vi "browseVariant.vi"(4 "Variant":variant caption="Value", 5 "Name":string, 6 "error in (no error)":errorcluster, 7 "ParentTag":string, 9 "VariantProbe.lvclass in":refnum<class "VariantTree__VP.lvclass">) -> (0 "error out":errorcluster, 3 "VariantProbe.lvclass out":refnum<class "VariantTree__VP.lvclass">)   [LabVIEW 2011, in "VariantTree__VP.lvclass"]
uses:
  VariantTree__VP.lvclass
  VariantTree__VP.lvclass/VariantTree__VP.ctl
  <vilib>/Utility/VariantDataType/VariantType.lvlib
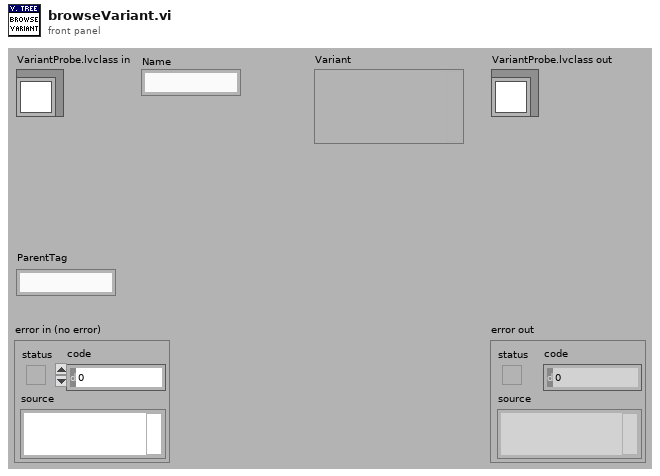
[diagram p1: front panel]
types:
  T1 = typedef "Type Descriptor Enumeration__ogtk.ctl" = enum8{"<Null>", "I8", "I16", "I32", "I64", "U8", "U16", "U32", "U64", "SGL", "DBL", "EXT", "CSG", "CDB", "CXT", "0x0F", "0x10", "0x11", "0x12", "0x13", "0x14", "Enum U8", "Enum U16", "Enum U32", "Enum U64", "SGL PQ", "DBL PQ", "EXT PQ", "CSG PQ", "CDB PQ", "CXT PQ", "0x1F", "0x20", "Boolean", "0x22", "0x23", "0x24", "0x25", "0x26", "0x27", "0x28", "0x29", "0x2A", "0x2B", "0x2C", "0x2D", "0x2E", "0x2F", "String", "0x31", "Path", "Pict", "0x34", "0x35", "0x36", "DAQ", "0x38", "0x39", "0x3A", "0x3B", "0x3C", "0x3D", "0x3E", "0x3F", "Array", "0x41", "0x42", "0x43", "0x44", "0x45", "0x46", "0x47", "0x48", "0x49", "0x4A", "0x4B", "0x4C", "0x4D", "0x4E", "0x4F", "Cluster", "0x51", "0x52", "Variant", "Waveform", "0x55", "0x56", "0x57", "0x58", "0x59", "0x5A", "0x5B", "0x5C", "0x5D", "0x5E", "0x5F", "0x60", "0x61", "0x62", "0x63", "0x64", "0x65", "0x66", "0x67", "0x68", "0x69", "0x6A", "0x6B", "0x6C", "0x6D", "0x6E", "0x6F", "Refnum"}
  T2 = typedef "Type Descriptor Header__ogtk.ctl" = cluster{"length":u16, "private":u8, "type":T1, "# elements":u16}
  T3 = typedef "Physical Units__ogtk.ctl" = cluster{"Base Units":enum16{"radian", "steradian", "second", "meter", "kilogram", "ampere", "kelvin", "mole", "candela"}, "Exponent":i16}
  T4 = enum16{"radian", "steradian", "second", "meter", "kilogram", "ampere", "kelvin", "mole", "candela"}
  T5 = typedef "VariantType.lvlib/RefnumType.ctl" = enum16{"NotARefnum", "UnknownRefnum", "Generic", "Datalog", "ByteStream", "Device", "Occurence", "TCPNetConnection", "Auto", "Menu", "Imaq", "Hardware", "DataSocket", "Visa", "IVI", "UDPNetConnection", "Notifier", "Queue", "Irda", "EventReg", "DotNet", "UserEvent", "Callback", "UNUSED_EMPTY_POSITION", "BlueToothNetConnection", "LVObjApp", "LVObjVI", "LVObjUnknown", "GenericClass", "UserDefinedRefnumTag", "DataValue"}
  T6 = enum32{"invalid VI type", "Standard VI", "Control VI", "Global VI", "Polymorphic VI", "Configuration VI", "SubSystem", "Facade VI", "Method VI", "Statechart Diagram VI"}
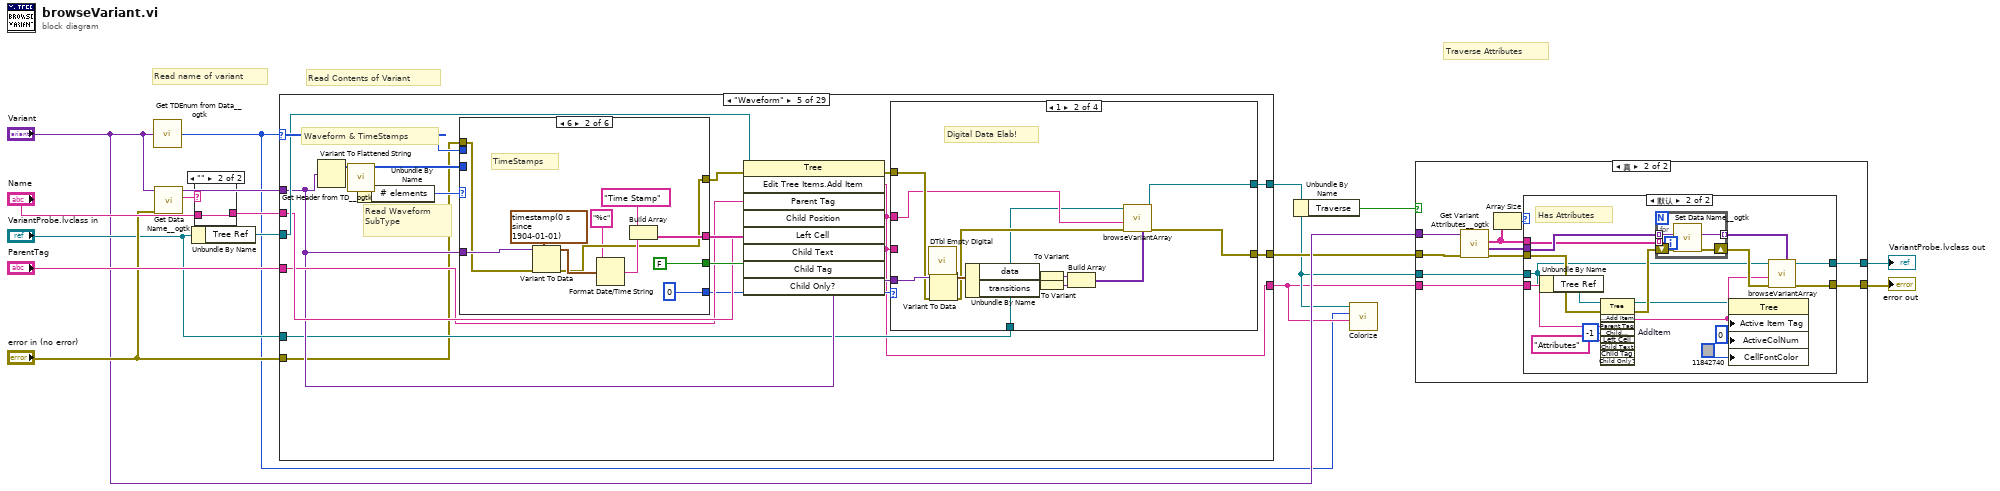
[diagram p0: block diagram]
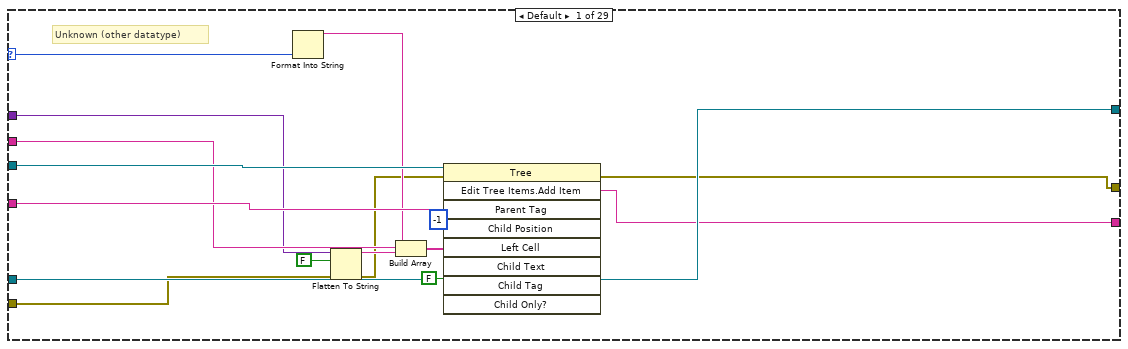
[diagram p5: hidden frame]
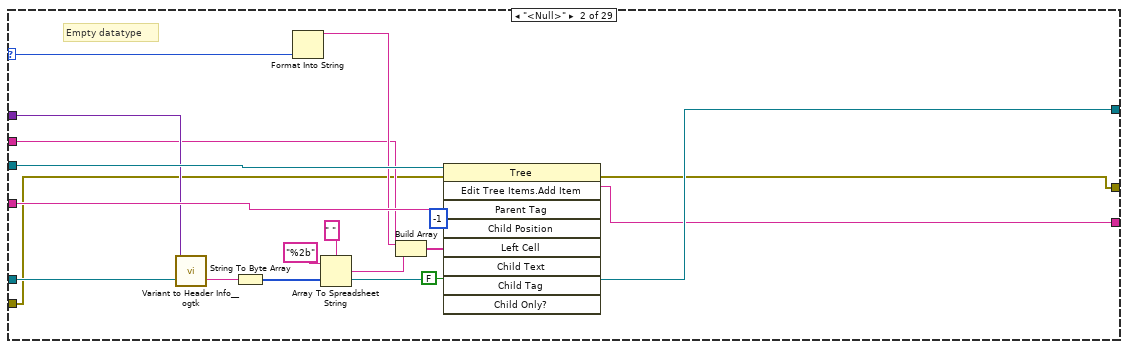
[diagram p6: hidden frame]
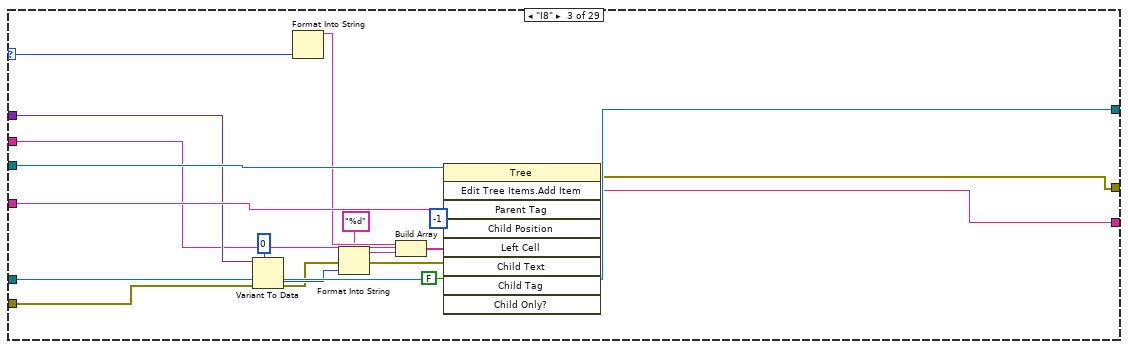
[diagram p7: hidden frame]
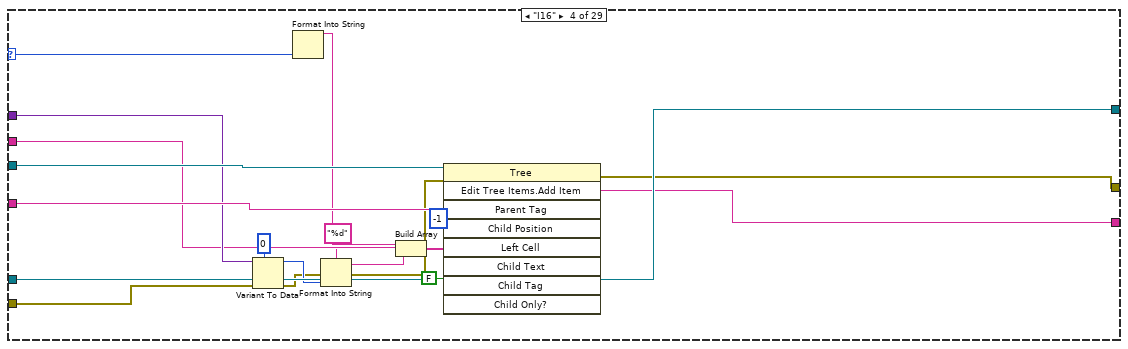
[diagram p8: hidden frame]
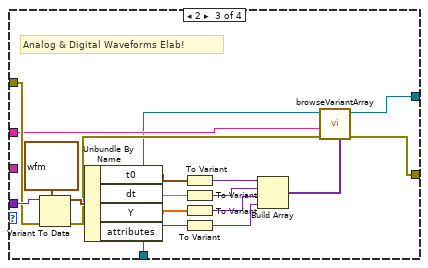
[diagram p10: hidden frame]
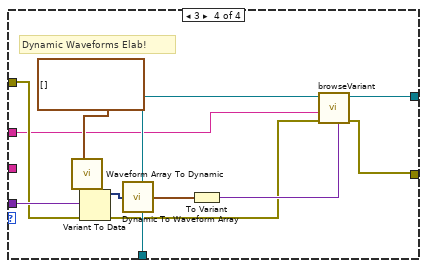
[diagram p11: hidden frame]
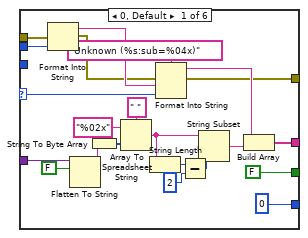
[diagram p12: hidden frame]
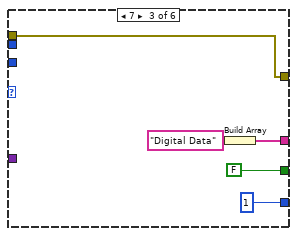
[diagram p13: hidden frame]
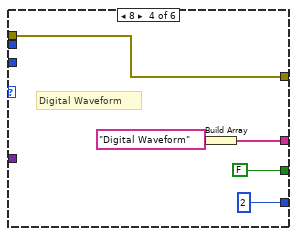
[diagram p14: hidden frame]
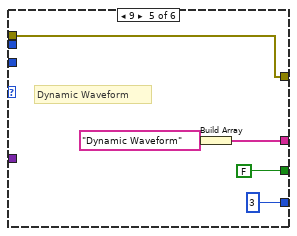
[diagram p15: hidden frame]
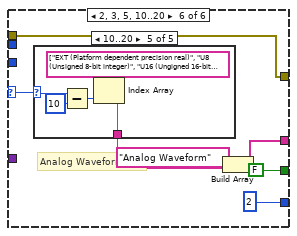
[diagram p16: hidden frame]
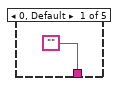
[diagram p17: hidden frame]
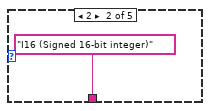
[diagram p18: hidden frame]
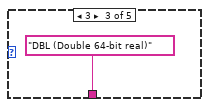
[diagram p19: hidden frame]
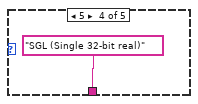
[diagram p20: hidden frame]
diagram:
  # "Traverse Attributes"
  # "Read Contents of Variant"
  # "Read name of variant"
  n1 = call <userlib>:"Get TDEnum from Data__ogtk.vi"("Data"="Variant") -> ("Type Descriptor Enumeration"=w1:T1)  [unwired: 4 in]
  n2 = call <userlib>:"Get Data Name__ogtk.vi"("error in (no error)"="error in (no error)", "Data"="Variant") -> ("Data Name"=w16:string, "Data dup"=w14:variant)  [unwired: 7 in, 1 out]
  n3 = Unbundle By Name("VariantProbe.lvclass in") -> ("Tree Ref"=w4:refnum<vi>)
  n4 = case shown="\"\"" w16 {
    selector: w16 -> [w17 _]
    tunnel: [w17 w18] -> w13
    tunnel: "Name" -> [_ w18]
    frame Default {
    }
    frame "" {
    }
  }
  n5 = case shown="\"Waveform\"" w1 {
    selector: w1 -> [w34 w52 w71 w90 w105 w237 w256 w275 w294 w313 w332 w350 w368 w386 w404 w422 w440 w463 w497 w531 w565 w591 w607 w624 w640 _ _ _ w711]
    tunnel: w14 -> [w25 w41 w64 w83 w97 w230 w249 w268 w287 w306 w325 w339 w358 w376 w394 w412 w430 w468 w485 w519 w553 w580 w598 w615 w631 w652 w666 w696 w702]
    tunnel: w4 -> [w31 w49 w68 w87 w104 w234 w253 w272 w291 w310 w329 w347 w365 w383 w401 w419 w437 w467 w494 w528 w562 w588 w604 w621 w637 w662 w677 w701 w709]
    tunnel: "ParentTag" -> [w33 w51 w70 w89 w99 w236 w255 w274 w293 w312 w331 w349 w367 w385 w403 w421 w439 w466 w496 w530 w564 w590 w606 w623 w639 w661 w676 w700 w710]
    tunnel: w13 -> [w26 w40 w63 w82 w100 w229 w248 w267 w286 w305 w324 w340 w357 w375 w393 w411 w429 w449 w488 w522 w556 w579 w599 w614 w632 w653 w673 w695 w707]
    tunnel: "VariantProbe.lvclass in" -> [w23 w38 w61 w80 w96 w227 w246 w265 w284 w303 w322 w337 w355 w373 w391 w409 w427 w445 w478 w512 w546 w577 w596 w612 w629 w643 w671 w690 w706]
    tunnel: [w23 w38 w61 w80 w95 w227 w246 w265 w284 w303 w322 w337 w355 w373 w391 w409 w427 w445 w478 w512 w546 w577 w596 w612 w629 w642 w670 w688 w706] -> w3
    tunnel: "error in (no error)" -> [w22 w37 w59 w78 w94 w226 w244 w264 w283 w301 w321 w335 w354 w372 w390 w408 w425 w444 w477 w511 w545 w575 w594 w609 w628 w649 w668 w693 _]
    tunnel: [w20 w36 w60 w79 w92 w225 w245 w263 w282 w302 w314 w334 w352 w370 w388 w406 w424 w442 w472 w506 w540 w574 w593 w611 w626 w646 w669 w692 w705] -> w8
    tunnel: [w19 w35 w53 w72 w91 w219 w238 w257 w276 w295 w315 w333 w351 w369 w387 w405 w423 w441 w471 w505 w539 w573 w592 w608 w625 w641 w667 w687 w704] -> w2
    frame Default {
      # "Unknown (other datatype)"
      n6 = Format Into String(w34) -> (resulting string=w30:string)  [unwired: 3 in, 1 out]
      n7 = Flatten To String(anything=w25, prepend array or string size? (T)=FALSE, error in (no error)=w22) -> (data string=w28:string, error out=w21:errorcluster)  [unwired: 1 in, 1 out]
      n8 = Build Array(w30, w28) -> (w29:string[])
      n9 = invoke class="Tree" method="Edit Tree Items.Add Item"(reference=w31, error in=w21, "Parent Tag"=w33, "Child Position"=-1, "Left Cell"=w26, "Child Text"=w29, "Child Only?"=FALSE) -> (error out=w20:errorcluster, "Edit Tree Items:Add Item"=w19:string)  [unwired: 2 in, 7 out]
    }
    frame "<Null>" {
      # "Empty datatype"
      n10 = call <userlib>:"Variant to Header Info__ogtk.vi"("Variant"=w41) -> ("data string"=w43:string)  [unwired: 3 in, 2 out]
      n11 = String To Byte Array(string=w43) -> (unsigned byte array=w42:u8[])
      n12 = Format Into String(w52) -> (resulting string=w48:string)  [unwired: 3 in, 1 out]
      n13 = Array To Spreadsheet String(delimiter (Tab)=" ", array=w42, 3:"%2b" ("format string")) -> (spreadsheet string=w44:string)
      n14 = Build Array(w48, w44) -> (w47:string[])
      n15 = invoke class="Tree" method="Edit Tree Items.Add Item"(reference=w49, error in=w37, "Parent Tag"=w51, "Child Position"=-1, "Left Cell"=w40, "Child Text"=w47, "Child Only?"=FALSE) -> (error out=w36:errorcluster, "Edit Tree Items:Add Item"=w35:string)  [unwired: 2 in, 7 out]
    }
    frame "I8" {
      n16 = Variant To Data(error in=w59, type=i8 0, Variant=w64) -> (data=w58:i8, error out=w55:errorcluster)
      n17 = Format Into String(w71) -> (resulting string=w67:string)  [unwired: 3 in, 1 out]
      n18 = Format Into String(format string="%d", error in=w55, w58) -> (resulting string=w57:string, error out=w54:errorcluster)  [unwired: 1 in]
      n19 = Build Array(w67, w57) -> (w66:string[])
      n20 = invoke class="Tree" method="Edit Tree Items.Add Item"(reference=w68, error in=w54, "Parent Tag"=w70, "Child Position"=-1, "Left Cell"=w63, "Child Text"=w66, "Child Only?"=FALSE) -> (error out=w60:errorcluster, "Edit Tree Items:Add Item"=w53:string)  [unwired: 2 in, 7 out]
    }
    frame "I16" {
      n21 = Variant To Data(error in=w78, type=i16 0, Variant=w83) -> (data=w76:i16, error out=w75:errorcluster)
      n22 = Format Into String(w90) -> (resulting string=w86:string)  [unwired: 3 in, 1 out]
      n23 = Format Into String(format string="%d", error in=w75, w76) -> (resulting string=w73:string, error out=w74:errorcluster)  [unwired: 1 in]
      n24 = Build Array(w86, w73) -> (w85:string[])
      n25 = invoke class="Tree" method="Edit Tree Items.Add Item"(reference=w87, error in=w74, "Parent Tag"=w89, "Child Position"=-1, "Left Cell"=w82, "Child Text"=w85, "Child Only?"=FALSE) -> (error out=w79:errorcluster, "Edit Tree Items:Add Item"=w72:string)  [unwired: 2 in, 7 out]
    }
    frame "Waveform" {
      # "Read Waveform\nSubType"
      # "Waveform & TimeStamps"
      n26 = Variant To Flattened String(Variant=w97) -> (1:w108:i16[])  [unwired: 1 out]
      n27 = call <userlib>:"Get Header from TD__ogtk.vi"("Type Descriptor"=w108) -> ("Type Descriptor Header"=w106:T2)
      n28 = Unbundle By Name(w106) -> ("# elements"=w107:u16)
      n29 = case shown="6" w107 {
        selector: w107 -> [w163 _ _ _ _ w208]
        tunnel: [w165 w184 w191 w196 w201 w209] -> w102
        tunnel: w97 -> [w164 w186 _ _ _ _]
        tunnel: w108 -> [_ _ _ _ _ _]
        tunnel: [0 0 1 2 3 2] -> w98
        tunnel: [FALSE ("Child Only?") FALSE ("Child Only?") FALSE ("Child Only?") FALSE ("Child Only?") FALSE ("Child Only?") FALSE ("Child Only?")] -> w101
        tunnel: w105 -> [w159 _ _ _ _ _]
        tunnel: [w157 w178 w188 w193 w198 w203] -> w103
        tunnel: w94 -> [w155 w181 w188 w193 w198 w203]
        frame 0, Default {
          n30 = Format Into String(error in=w155, w159) -> (resulting string=w158:string, error out=w156:errorcluster)  [unwired: 2 in]
          n31 = Flatten To String(anything=w164, prepend array or string size? (T)=FALSE) -> (data string=w166:string)  [unwired: 2 in, 2 out]
          n32 = String To Byte Array(string=w166) -> (unsigned byte array=w160:u8[])
          n33 = Array To Spreadsheet String(delimiter (Tab)=" ", array=w160, 3:"%02x" ("format string")) -> (spreadsheet string=w172:string)
          n34 = String Length(string=w172) -> (length=w173:i32)
          n35 = Format Into String(format string="Unknown (%s:sub=%04x)", error in=w156, w158, w163) -> (resulting string=w169:string, error out=w157:errorcluster)  [unwired: 1 in]
          n36 = Subtract(x=w173, y=2) -> (x-y=w175:i32)
          n37 = String Subset(string=w172, length (rest)=w175) -> (substring=w176:string)  [unwired: 1 in]
          n38 = Build Array(w169, w176) -> (w165:string[])
        }
        frame 6 {
          # "TimeStamps"
          n39 = Variant To Data(error in=w181, type=timestamp(0 s since 1904-01-01), Variant=w186) -> (data=w179:timestamp, error out=w178:errorcluster)
          n40 = Format Date/Time String(time format string (%c)="%c" ("format string"), seconds (now)=w179) -> (date/time string=w180:string)  [unwired: 1 in]
          n41 = Build Array("Time Stamp" ("format string"), w180) -> (w184:string[])
        }
        frame 7 {
          n42 = Build Array("Digital Data" ("format string")) -> (w191:string[])
        }
        frame 8 {
          # "Digital Waveform"
          n43 = Build Array("Digital Waveform" ("format string")) -> (w196:string[])
        }
        frame 9 {
          # "Dynamic Waveform"
          n44 = Build Array("Dynamic Waveform" ("format string")) -> (w201:string[])
        }
        frame 2, 3, 5, 10..20 {
          # "Analog Waveform"
          n45 = case shown="10..20" w208 {
            selector: w208 -> [_ _ _ _ w216]
            tunnel: ["" "I16 (Signed 16-bit integer)" "DBL (Double 64-bit real)" "SGL (Single 32-bit real)" w218] -> w204
            frame 0, Default {
            }
            frame 2 {
            }
            frame 3 {
            }
            frame 5 {
            }
            frame 10..20 {
              n46 = Subtract(x=w216, y=u16 10) -> (x-y=w214:u16)
              n47 = Index Array(array=string[] ["EXT (Platform dependent precision real)", "U8 (Unsigned 8-bit integer)", "U16 (Ungigned 16-bit integer)", "U32 (Unsigned 32-bit integer)", "I8 (Signed 8-bit integer)", "I32 (Signed 32-bit integer)", "CSG (Single 32-bit complex real)", "CDB (Double 64-bit complex real)", "CXT (Extended complex real)", "I64 (Signed 64-bit integer)", "U64 (Unsigned 64-bit integer)"], index=w214) -> (element=w218:string)
            }
          }
          n48 = Build Array("Analog Waveform" ("format string"), w204) -> (w209:string[])
        }
      }
      n49 = invoke class="Tree" method="Edit Tree Items.Add Item"(reference=w104, error in=w103, "Parent Tag"=w99, "Left Cell"=w100, "Child Text"=w102, "Child Only?"=w101) -> (error out=w93:errorcluster, "Edit Tree Items:Add Item"=w91:string)  [unwired: 3 in, 7 out]
      n50 = case shown="1" w98 {
        tunnel: w91 -> [_ w114 w128 w147]
        tunnel: w97 -> [_ w124 w142 w150]
        tunnel: w91 -> [_ _ _ _]
        tunnel: w96 -> [w110 w112 w126 w148]
        tunnel: [w110 w111 w125 w145] -> w95
        tunnel: w93 -> [w109 w117 w131 w149]
        tunnel: [w109 w113 w127 w144] -> w92
        frame 0, Default {
          # "No further elaborations!"
        }
        frame 1 {
          # "Digital Data Elab!"
          n51 = call <vilib>:"DTbl Empty Digital.vi"() -> ("digital data"=w123:digitaldata)  [unwired: 5 in]
          n52 = Variant To Data(error in=w117, type=w123, Variant=w124) -> (data=w122:digitaldata, error out=w116:errorcluster)
          n53 = Unbundle By Name(w122) -> ("data"=w119:u8[][], "transitions"=w118:u32[])
          n54 = To Variant(anything=w119) -> (Variant=w121:variant)
          n55 = To Variant(anything=w118) -> (Variant=w120:variant)
          n56 = Build Array(w121, w120) -> (w115:variant[])
          n57 = call-dynamic "browseVariantArray.vi"("Array of Variants"=w115, "error in"=w116, "ParentTag"=w114, "VariantProbe.lvclass in"=w112) -> ("error out"=w113:errorcluster, "VariantProbe.lvclass out"=w111:refnum<class "VariantTree__VP.lvclass">)  [unwired: 4 in]
        }
        frame 2 {
          # "Analog & Digital Waveforms Elab!"
          n58 = Variant To Data(error in=w131, type=waveform(dbl) {"t0"=timestamp(0 s since 1904-01-01), "dt"=1.0, "Y"=[]} ("waveform"), Variant=w142) -> (data=w134:waveform(dbl), error out=w129:errorcluster)
          n59 = Unbundle By Name(w134) -> ("t0"=w136:timestamp, "dt"=w138:dbl, "Y"=w137:dbl[], "attributes"=w133:variant)
          n60 = To Variant(anything=w136) -> (Variant=w135:variant)
          n61 = To Variant(anything=w138) -> (Variant=w140:variant)
          n62 = To Variant(anything=w137) -> (Variant=w139:variant)
          n63 = To Variant(anything=w133) -> (Variant=w132:variant)
          n64 = Build Array(w135, w140, w139, w132) -> (w130:variant[])
          n65 = call-dynamic "browseVariantArray.vi"("Array of Variants"=w130, "error in"=w129, "ParentTag"=w128, "VariantProbe.lvclass in"=w126) -> ("error out"=w127:errorcluster, "VariantProbe.lvclass out"=w125:refnum<class "VariantTree__VP.lvclass">)  [unwired: 4 in]
        }
        frame 3 {
          # "Dynamic Waveforms Elab!"
          n66 = call <vilib>:"Waveform Array To Dynamic.vi"("Input"=waveform(dbl)[] []) -> ("Output"=w154:dynamicdata)  [unwired: 4 in]
          n67 = Variant To Data(error in=w149, type=w154, Variant=w150) -> (data=w153:dynamicdata, error out=w143:errorcluster)
          n68 = call <vilib>:"Dynamic To Waveform Array.vi"("Input"=w153) -> ("Output"=w151:waveform(dbl)[])  [unwired: 4 in]
          n69 = To Variant(anything=w151) -> (Variant=w146:variant)
          n70 = call-dynamic "browseVariant.vi"("Variant"=w146, "error in (no error)"=w143, "ParentTag"=w147, "VariantProbe.lvclass in"=w148) -> ("error out"=w144:errorcluster, "VariantProbe.lvclass out"=w145:refnum<class "VariantTree__VP.lvclass">)  [unwired: 4 in]
        }
      }
    }
    frame "I32" {
      n71 = Variant To Data(error in=w226, type=0, Variant=w230) -> (data=w222:i32, error out=w223:errorcluster)
      n72 = Format Into String(w237) -> (resulting string=w233:string)  [unwired: 3 in, 1 out]
      n73 = Format Into String(format string="%d", error in=w223, w222) -> (resulting string=w220:string, error out=w221:errorcluster)  [unwired: 1 in]
      n74 = Build Array(w233, w220) -> (w232:string[])
      n75 = invoke class="Tree" method="Edit Tree Items.Add Item"(reference=w234, error in=w221, "Parent Tag"=w236, "Child Position"=-1, "Left Cell"=w229, "Child Text"=w232, "Child Only?"=FALSE) -> (error out=w225:errorcluster, "Edit Tree Items:Add Item"=w219:string)  [unwired: 2 in, 7 out]
    }
    frame "I64" {
      # "I64"
      n76 = Variant To Data(error in=w244, type=i64 0, Variant=w249) -> (data=w241:i64, error out=w242:errorcluster)
      n77 = Format Into String(w256) -> (resulting string=w252:string)  [unwired: 3 in, 1 out]
      n78 = Format Into String(format string="%d", error in=w242, w241) -> (resulting string=w240:string, error out=w239:errorcluster)  [unwired: 1 in]
      n79 = Build Array(w252, w240) -> (w251:string[])
      n80 = invoke class="Tree" method="Edit Tree Items.Add Item"(reference=w253, error in=w239, "Parent Tag"=w255, "Child Position"=-1, "Left Cell"=w248, "Child Text"=w251, "Child Only?"=FALSE) -> (error out=w245:errorcluster, "Edit Tree Items:Add Item"=w238:string)  [unwired: 2 in, 7 out]
    }
    frame "U8" {
      n81 = Variant To Data(error in=w264, type=u8 0, Variant=w268) -> (data=w261:u8, error out=w260:errorcluster)
      n82 = Format Into String(w275) -> (resulting string=w271:string)  [unwired: 3 in, 1 out]
      n83 = Format Into String(format string="%d", error in=w260, w261) -> (resulting string=w258:string, error out=w259:errorcluster)  [unwired: 1 in]
      n84 = Build Array(w271, w258) -> (w270:string[])
      n85 = invoke class="Tree" method="Edit Tree Items.Add Item"(reference=w272, error in=w259, "Parent Tag"=w274, "Child Position"=-1, "Left Cell"=w267, "Child Text"=w270, "Child Only?"=FALSE) -> (error out=w263:errorcluster, "Edit Tree Items:Add Item"=w257:string)  [unwired: 2 in, 7 out]
    }
    frame "U16" {
      n86 = Variant To Data(error in=w283, type=u16 0, Variant=w287) -> (data=w277:u16, error out=w278:errorcluster)
      n87 = Format Into String(w294) -> (resulting string=w290:string)  [unwired: 3 in, 1 out]
      n88 = Format Into String(format string="%d", error in=w278, w277) -> (resulting string=w280:string, error out=w279:errorcluster)  [unwired: 1 in]
      n89 = Build Array(w290, w280) -> (w289:string[])
      n90 = invoke class="Tree" method="Edit Tree Items.Add Item"(reference=w291, error in=w279, "Parent Tag"=w293, "Child Position"=-1, "Left Cell"=w286, "Child Text"=w289, "Child Only?"=FALSE) -> (error out=w282:errorcluster, "Edit Tree Items:Add Item"=w276:string)  [unwired: 2 in, 7 out]
    }
    frame "U32" {
      n91 = Variant To Data(error in=w301, type=u32 0, Variant=w306) -> (data=w299:u32, error out=w298:errorcluster)
      n92 = Format Into String(w313) -> (resulting string=w309:string)  [unwired: 3 in, 1 out]
      n93 = Format Into String(format string="%d", error in=w298, w299) -> (resulting string=w296:string, error out=w297:errorcluster)  [unwired: 1 in]
      n94 = Build Array(w309, w296) -> (w308:string[])
      n95 = invoke class="Tree" method="Edit Tree Items.Add Item"(reference=w310, error in=w297, "Parent Tag"=w312, "Child Position"=-1, "Left Cell"=w305, "Child Text"=w308, "Child Only?"=FALSE) -> (error out=w302:errorcluster, "Edit Tree Items:Add Item"=w295:string)  [unwired: 2 in, 7 out]
    }
    frame "U64" {
      # "U64"
      n96 = Variant To Data(error in=w321, type=u64 0, Variant=w325) -> (data=w319:u64, error out=w318:errorcluster)
      n97 = Format Into String(w332) -> (resulting string=w328:string)  [unwired: 3 in, 1 out]
      n98 = Format Into String(format string="%d", error in=w318, w319) -> (resulting string=w316:string, error out=w317:errorcluster)  [unwired: 1 in]
      n99 = Build Array(w328, w316) -> (w327:string[])
      n100 = invoke class="Tree" method="Edit Tree Items.Add Item"(reference=w329, error in=w317, "Parent Tag"=w331, "Child Position"=-1, "Left Cell"=w324, "Child Text"=w327, "Child Only?"=FALSE) -> (error out=w314:errorcluster, "Edit Tree Items:Add Item"=w315:string)  [unwired: 2 in, 7 out]
    }
    frame "SGL" {
      n101 = Variant To Data(error in=w335, type=sgl 0.0, Variant=w339) -> (data=w342:sgl, error out=w336:errorcluster)
      n102 = Format Into String(w350) -> (resulting string=w346:string)  [unwired: 3 in, 1 out]
      n103 = Format Value(format string="%f", value (0)=w342) -> (output string=w341:string)  [unwired: 1 in]
      n104 = Build Array(w346, w341) -> (w345:string[])
      n105 = invoke class="Tree" method="Edit Tree Items.Add Item"(reference=w347, error in=w336, "Parent Tag"=w349, "Child Position"=-1, "Left Cell"=w340, "Child Text"=w345, "Child Only?"=FALSE) -> (error out=w334:errorcluster, "Edit Tree Items:Add Item"=w333:string)  [unwired: 2 in, 7 out]
    }
    frame "DBL" {
      n106 = Variant To Data(error in=w354, type=0.0, Variant=w358) -> (data=w360:dbl, error out=w353:errorcluster)
      n107 = Format Into String(w368) -> (resulting string=w364:string)  [unwired: 3 in, 1 out]
      n108 = Format Value(format string="%f", value (0)=w360) -> (output string=w359:string)  [unwired: 1 in]
      n109 = Build Array(w364, w359) -> (w363:string[])
      n110 = invoke class="Tree" method="Edit Tree Items.Add Item"(reference=w365, error in=w353, "Parent Tag"=w367, "Child Position"=-1, "Left Cell"=w357, "Child Text"=w363, "Child Only?"=FALSE) -> (error out=w352:errorcluster, "Edit Tree Items:Add Item"=w351:string)  [unwired: 2 in, 7 out]
    }
    frame "EXT" {
      n111 = Variant To Data(error in=w372, type=ext 0.0, Variant=w376) -> (data=w378:ext, error out=w371:errorcluster)
      n112 = Format Into String(w386) -> (resulting string=w382:string)  [unwired: 3 in, 1 out]
      n113 = Format Value(format string="%f", value (0)=w378) -> (output string=w377:string)  [unwired: 1 in]
      n114 = Build Array(w382, w377) -> (w381:string[])
      n115 = invoke class="Tree" method="Edit Tree Items.Add Item"(reference=w383, error in=w371, "Parent Tag"=w385, "Child Position"=-1, "Left Cell"=w375, "Child Text"=w381, "Child Only?"=FALSE) -> (error out=w370:errorcluster, "Edit Tree Items:Add Item"=w369:string)  [unwired: 2 in, 7 out]
    }
    frame "CSG" {
      n116 = Variant To Data(error in=w390, type=csg 0.0+0.0i, Variant=w394) -> (data=w396:csg, error out=w389:errorcluster)
      n117 = Format Into String(w404) -> (resulting string=w400:string)  [unwired: 3 in, 1 out]
      n118 = Format Value(format string="%f", value (0)=w396) -> (output string=w395:string)  [unwired: 1 in]
      n119 = Build Array(w400, w395) -> (w399:string[])
      n120 = invoke class="Tree" method="Edit Tree Items.Add Item"(reference=w401, error in=w389, "Parent Tag"=w403, "Child Position"=-1, "Left Cell"=w393, "Child Text"=w399, "Child Only?"=FALSE) -> (error out=w388:errorcluster, "Edit Tree Items:Add Item"=w387:string)  [unwired: 2 in, 7 out]
    }
    frame "CDB" {
      n121 = Variant To Data(error in=w408, type=cdb 0.0+0.0i, Variant=w412) -> (data=w414:cdb, error out=w407:errorcluster)
      n122 = Format Into String(w422) -> (resulting string=w418:string)  [unwired: 3 in, 1 out]
      n123 = Format Value(format string="%f", value (0)=w414) -> (output string=w413:string)  [unwired: 1 in]
      n124 = Build Array(w418, w413) -> (w417:string[])
      n125 = invoke class="Tree" method="Edit Tree Items.Add Item"(reference=w419, error in=w407, "Parent Tag"=w421, "Child Position"=-1, "Left Cell"=w411, "Child Text"=w417, "Child Only?"=FALSE) -> (error out=w406:errorcluster, "Edit Tree Items:Add Item"=w405:string)  [unwired: 2 in, 7 out]
    }
    frame "CXT" {
      n126 = Variant To Data(error in=w425, type=cxt 0.0+0.0i, Variant=w430) -> (data=w432:cxt, error out=w426:errorcluster)
      n127 = Format Into String(w440) -> (resulting string=w436:string)  [unwired: 3 in, 1 out]
      n128 = Format Value(format string="%f", value (0)=w432) -> (output string=w431:string)  [unwired: 1 in]
      n129 = Build Array(w436, w431) -> (w435:string[])
      n130 = invoke class="Tree" method="Edit Tree Items.Add Item"(reference=w437, error in=w426, "Parent Tag"=w439, "Child Position"=-1, "Left Cell"=w429, "Child Text"=w435, "Child Only?"=FALSE) -> (error out=w424:errorcluster, "Edit Tree Items:Add Item"=w423:string)  [unwired: 2 in, 7 out]
    }
    frame "Enum U8".."Enum U64" {
      # "Make a string with all the possible values of the enum"
      n131 = call <userlib>:"Get Strings from Enum__ogtk.vi"("error in (no error)"=w444, "Enum"=w468) -> ("error out"=w443:errorcluster, "String Value"=w462:string, "Enum Strings"=w461:string[], "Enum Name"=w450:string)  [unwired: 6 in]
      n132 = Format Into String(w463) -> (resulting string=w459:string)  [unwired: 3 in, 1 out]
      n133 = case shown="\"\"" w450 {
        selector: w450 -> [w469 _]
        tunnel: [w469 w470] -> w448
        tunnel: w449 -> [_ w470]
        frame Default {
        }
        frame "" {
        }
      }
      n134 = Array To Spreadsheet String(delimiter (Tab)=", ", array=w461, 3:"%s" ("format string")) -> (spreadsheet string=w452:string)
      n135 = Search and Replace String(replace all?=TRUE ("replace all? (F)"), input string=w452, search string="\r\n") -> (result string=w451:string)  [unwired: 5 in, 3 out]
      n136 = Concatenate Strings(w459, " " ("string"), "(" ("string"), w451, ")" ("string")) -> (w446:string)
      n137 = Build Array(w446, w462) -> (w464:string[])
      n138 = invoke class="Tree" method="Edit Tree Items.Add Item"(reference=w467, error in=w443, "Parent Tag"=w466, "Child Position"=-1, "Left Cell"=w448, "Child Text"=w464, "Child Only?"=FALSE) -> (error out=w442:errorcluster, "Edit Tree Items:Add Item"=w441:string)  [unwired: 2 in, 7 out]
    }
    frame "SGL PQ" {
      # "strip last '*'"
      # "Add physical quantity to string"
      n139 = call <userlib>:"Get Physical Units__ogtk.vi"("error in (no error)"=w477, "Float or Array of Floats"=w485) -> ("error out"=w476:errorcluster, "Physical Units"=w484:T3[])  [unwired: 8 in]
      n140 = call <userlib>:"Strip Units__ogtk.vi"("error in (no error)"=w476, "Number or 1D array with units"=w485) -> ("error out"=w475:errorcluster, "Pure Number(s) (base units)"=w486:variant)  [unwired: 8 in]
      n141 = for {
        tunnel: w484 -> [w504] mode=indexing
        tunnel: [w500] -> w483 mode=indexing
        shift-right: [w498] -> w474
        shift-left: w475 -> [w499]
        n142 = Unbundle(w504) -> ("Base Units"=w503:T4, "Exponent"=w502:i16)
        n143 = Format Into String(format string="%s ^(%d)*", error in=w499, w503, w502) -> (resulting string=w500:string, error out=w498:errorcluster)  [unwired: 1 in]
      }
      n144 = Format Into String(w497) -> (resulting string=w493:string)  [unwired: 3 in, 1 out]
      n145 = Variant To Data(error in=w474, type=sgl 0.0, Variant=w486) -> (data=w489:sgl, error out=w473:errorcluster)
      n146 = Format Value(format string="%f", value (0)=w489) -> (output string=w480:string)  [unwired: 1 in]
      n147 = Concatenate Strings(w480, w483) -> (w482:string)
      n148 = call <userlib>:"Slice String__ogtk.vi"("slice"=":-1", "string"=w482) -> ("substring"=w479:string)  [unwired: 5 in]
      n149 = Build Array(w493, w479) -> (w492:string[])
      n150 = invoke class="Tree" method="Edit Tree Items.Add Item"(reference=w494, error in=w473, "Parent Tag"=w496, "Child Position"=-1, "Left Cell"=w488, "Child Text"=w492, "Child Only?"=FALSE) -> (error out=w472:errorcluster, "Edit Tree Items:Add Item"=w471:string)  [unwired: 2 in, 7 out]
    }
    frame "DBL PQ" {
      # "strip last '*'"
      # "Add physical quantity to string"
      n151 = call <userlib>:"Get Physical Units__ogtk.vi"("error in (no error)"=w511, "Float or Array of Floats"=w519) -> ("error out"=w510:errorcluster, "Physical Units"=w518:T3[])  [unwired: 8 in]
      n152 = call <userlib>:"Strip Units__ogtk.vi"("error in (no error)"=w510, "Number or 1D array with units"=w519) -> ("error out"=w509:errorcluster, "Pure Number(s) (base units)"=w520:variant)  [unwired: 8 in]
      n153 = for {
        tunnel: w518 -> [w538] mode=indexing
        tunnel: [w534] -> w517 mode=indexing
        shift-right: [w532] -> w508
        shift-left: w509 -> [w533]
        n154 = Unbundle(w538) -> ("Base Units"=w537:T4, "Exponent"=w536:i16)
        n155 = Format Into String(format string="%s ^(%d)*", error in=w533, w537, w536) -> (resulting string=w534:string, error out=w532:errorcluster)  [unwired: 1 in]
      }
      n156 = Format Into String(w531) -> (resulting string=w527:string)  [unwired: 3 in, 1 out]
      n157 = Variant To Data(error in=w508, type=0.0, Variant=w520) -> (data=w523:dbl, error out=w507:errorcluster)
      n158 = Format Value(format string="%f", value (0)=w523) -> (output string=w514:string)  [unwired: 1 in]
      n159 = Concatenate Strings(w514, w517) -> (w516:string)
      n160 = call <userlib>:"Slice String__ogtk.vi"("slice"=":-1", "string"=w516) -> ("substring"=w513:string)  [unwired: 5 in]
      n161 = Build Array(w527, w513) -> (w526:string[])
      n162 = invoke class="Tree" method="Edit Tree Items.Add Item"(reference=w528, error in=w507, "Parent Tag"=w530, "Child Position"=-1, "Left Cell"=w522, "Child Text"=w526, "Child Only?"=FALSE) -> (error out=w506:errorcluster, "Edit Tree Items:Add Item"=w505:string)  [unwired: 2 in, 7 out]
    }
    frame "EXT PQ" {
      # "strip last '*'"
      # "Add physical quantity to string"
      n163 = call <userlib>:"Get Physical Units__ogtk.vi"("error in (no error)"=w545, "Float or Array of Floats"=w553) -> ("error out"=w544:errorcluster, "Physical Units"=w552:T3[])  [unwired: 8 in]
      n164 = call <userlib>:"Strip Units__ogtk.vi"("error in (no error)"=w544, "Number or 1D array with units"=w553) -> ("error out"=w543:errorcluster, "Pure Number(s) (base units)"=w554:variant)  [unwired: 8 in]
      n165 = for {
        tunnel: w552 -> [w572] mode=indexing
        tunnel: [w568] -> w551 mode=indexing
        shift-right: [w566] -> w542
        shift-left: w543 -> [w567]
        n166 = Unbundle(w572) -> ("Base Units"=w571:T4, "Exponent"=w570:i16)
        n167 = Format Into String(format string="%s ^(%d)*", error in=w567, w571, w570) -> (resulting string=w568:string, error out=w566:errorcluster)  [unwired: 1 in]
      }
      n168 = Format Into String(w565) -> (resulting string=w561:string)  [unwired: 3 in, 1 out]
      n169 = Variant To Data(error in=w542, type=ext 0.0, Variant=w554) -> (data=w557:ext, error out=w541:errorcluster)
      n170 = Format Value(format string="%f", value (0)=w557) -> (output string=w548:string)  [unwired: 1 in]
      n171 = Concatenate Strings(w548, w551) -> (w550:string)
      n172 = call <userlib>:"Slice String__ogtk.vi"("slice"=":-1", "string"=w550) -> ("substring"=w547:string)  [unwired: 5 in]
      n173 = Build Array(w561, w547) -> (w560:string[])
      n174 = invoke class="Tree" method="Edit Tree Items.Add Item"(reference=w562, error in=w541, "Parent Tag"=w564, "Child Position"=-1, "Left Cell"=w556, "Child Text"=w560, "Child Only?"=FALSE) -> (error out=w540:errorcluster, "Edit Tree Items:Add Item"=w539:string)  [unwired: 2 in, 7 out]
    }
    frame "Boolean" {
      n175 = Variant To Data(error in=w575, type=TRUE, Variant=w580) -> (data=w584:bool, error out=w576:errorcluster)
      n176 = Format Into String(w591) -> (resulting string=w587:string)  [unwired: 3 in, 1 out]
      n177 = Append True/False String(1:w584, 2:"False" ("false string"), 3:"True" ("true string")) -> (0:w583:string)  [unwired: 1 in]
      n178 = Build Array(w587, w583) -> (w586:string[])
      n179 = invoke class="Tree" method="Edit Tree Items.Add Item"(reference=w588, error in=w576, "Parent Tag"=w590, "Child Position"=-1, "Left Cell"=w579, "Child Text"=w586, "Child Only?"=FALSE) -> (error out=w574:errorcluster, "Edit Tree Items:Add Item"=w573:string)  [unwired: 2 in, 7 out]
    }
    frame "String", "DAQ" {
      n180 = Variant To Data(error in=w594, type="", Variant=w598) -> (data=w600:string, error out=w595:errorcluster)
      n181 = Format Into String(w607) -> (resulting string=w603:string)  [unwired: 3 in, 1 out]
      n182 = Build Array(w603, w600) -> (w602:string[])
      n183 = invoke class="Tree" method="Edit Tree Items.Add Item"(reference=w604, error in=w595, "Parent Tag"=w606, "Child Position"=-1, "Left Cell"=w599, "Child Text"=w602, "Child Only?"=FALSE) -> (error out=w593:errorcluster, "Edit Tree Items:Add Item"=w592:string)  [unwired: 2 in, 7 out]
    }
    frame "Path" {
      n184 = Variant To Data(error in=w609, type=path "", Variant=w615) -> (data=w617:path, error out=w610:errorcluster)
      n185 = Format Into String(w624) -> (resulting string=w620:string)  [unwired: 3 in, 1 out]
      n186 = Path To String(path=w617) -> (string=w616:string)
      n187 = Build Array(w620, w616) -> (w619:string[])
      n188 = invoke class="Tree" method="Edit Tree Items.Add Item"(reference=w621, error in=w610, "Parent Tag"=w623, "Child Position"=-1, "Left Cell"=w614, "Child Text"=w619, "Child Only?"=FALSE) -> (error out=w611:errorcluster, "Edit Tree Items:Add Item"=w608:string)  [unwired: 2 in, 7 out]
    }
    frame "Pict" {
      # "Add pict information in binary form"
      # "Unknown (other datatype)"
      n189 = Format Into String(w640) -> (resulting string=w636:string)  [unwired: 3 in, 1 out]
      n190 = Flatten To String(anything=w631, prepend array or string size? (T)=FALSE, error in (no error)=w628) -> (data string=w634:string, error out=w627:errorcluster)  [unwired: 1 in, 1 out]
      n191 = Build Array(w636, w634) -> (w635:string[])
      n192 = invoke class="Tree" method="Edit Tree Items.Add Item"(reference=w637, error in=w627, "Parent Tag"=w639, "Child Position"=-1, "Left Cell"=w632, "Child Text"=w635, "Child Only?"=FALSE) -> (error out=w626:errorcluster, "Edit Tree Items:Add Item"=w625:string)  [unwired: 2 in, 7 out]
    }
    frame "Array" {
      # "Load Same VI recursive, just one time"
      # "New branch for array"
      n193 = call <userlib>:"Reshape Array to 1D VArray__ogtk.vi"("error in (no error)"=w649, "MultiD Array"=w652) -> ("error out"=w648:errorcluster, "Size(s)"=w651:u32[], "1D VArray"=w650:variant)  [unwired: 7 in]
      n194 = Multiply Array Elements(1:w651) -> (0:w654:u32)
      n195 = Format Into String(format string="[%d]", initial string="Array", w654) -> (resulting string=w656:string)  [unwired: 1 in, 1 out]
      n196 = Build Array(w656) -> (w655:string[])
      n197 = invoke class="Tree" method="Edit Tree Items.Add Item"(reference=w662, error in=w648, "Parent Tag"=w661, "Child Position"=-1, "Left Cell"=w653, "Child Text"=w655, "Child Only?"=FALSE) -> (error out=w647:errorcluster, "Edit Tree Items:Add Item"=w641:string)  [unwired: 2 in, 7 out]
      n198 = call <userlib>:"Array to Array of VData__ogtk.vi"("error in (no error)"=w647, "MultiD Array"=w650) -> ("error out"=w645:errorcluster, "1D Array of Variants"=w644:variant[])  [unwired: 8 in]
      n199 = call-dynamic "browseVariantArray.vi"("Array of Variants"=w644, "error in"=w645, "ParentTag"=w641, "VariantProbe.lvclass in"=w643) -> ("error out"=w646:errorcluster, "VariantProbe.lvclass out"=w642:refnum<class "VariantTree__VP.lvclass">)  [unwired: 4 in]
    }
    frame "Cluster" {
      # "Load Same VI recursive"
      # "New branch for cluster"
      n200 = invoke class="Tree" method="Edit Tree Items.Add Item"(reference=w677, error in=w668, "Parent Tag"=w676, "Child Position"=-1, "Left Cell"=w673, "Child Text"=string[] ["Cluster"], "Child Only?"=FALSE) -> (error out=w665:errorcluster, "Edit Tree Items:Add Item"=w667:string)  [unwired: 2 in, 7 out]
      n201 = call <userlib>:"Cluster to Array of VData__ogtk.vi"("error in (no error)"=w665, "Cluster"=w666) -> ("error out"=w664:errorcluster, "Array of VData"=w663:variant[])  [unwired: 8 in]
      n202 = for {
        tunnel: w667 -> [w686]
        shift-right: [w684] -> w670
        shift-left: w671 -> [w685]
        shift-right: [w683] -> w669
        shift-left: w664 -> [w678]
        tunnel: w663 -> [w681] mode=indexing
        n203 = call <userlib>:"Get Data Name__ogtk.vi"("error in (no error)"=w678, "Data"=w681) -> ("error out"=w679:errorcluster, "Data Name"=w682:string, "Data dup"=w680:variant)  [unwired: 7 in]
        n204 = call-dynamic "browseVariant.vi"("Variant"=w680, "Name"=w682, "error in (no error)"=w679, "ParentTag"=w686, "VariantProbe.lvclass in"=w685) -> ("error out"=w683:errorcluster, "VariantProbe.lvclass out"=w684:refnum<class "VariantTree__VP.lvclass">)  [unwired: 3 in]
      }
    }
    frame "Variant" {
      # "New Branch for variant"
      # "Load Same VI recursive"
      n205 = call <userlib>:"Unwrap VVariant__ogtk.vi"("error in (no error)"=w693, "VVariant"=w696) -> ("error out"=w694:errorcluster, "Variant"=w689:variant)  [unwired: 8 in]
      n206 = invoke class="Tree" method="Edit Tree Items.Add Item"(reference=w701, error in=w694, "Parent Tag"=w700, "Child Position"=-1, "Left Cell"=w695, "Child Text"=string[] ["Variant"], "Child Only?"=FALSE) -> (error out=w691:errorcluster, "Edit Tree Items:Add Item"=w687:string)  [unwired: 2 in, 7 out]
      n207 = call-dynamic "browseVariant.vi"("Variant"=w689, "error in (no error)"=w691, "ParentTag"=w687, "VariantProbe.lvclass in"=w690) -> ("error out"=w692:errorcluster, "VariantProbe.lvclass out"=w688:refnum<class "VariantTree__VP.lvclass">)  [unwired: 4 in]
    }
    frame "Refnum" {
      n208 = call <vilib>:"GetRefnumInfo.vi"("Variant"=w702) -> ("ReferenceType"=w703:T5)  [unwired: 7 in, 3 out]
      n209 = Format Into String(w711) -> (resulting string=w708:string)  [unwired: 3 in, 1 out]
      n210 = case shown="\"GenericClass\"" w703 {
        tunnel: w710 -> [w727 w739 w756 w772 w786]
        tunnel: w709 -> [w725 w737 w754 w770 w784]
        tunnel: w708 -> [w724 w736 w753 w769 w783]
        tunnel: w707 -> [w722 w734 w751 w767 w781]
        tunnel: [w718 w730 w747 w763 w777] -> w705
        tunnel: [w717 w729 w746 w762 w776] -> w704
        tunnel: w703 -> [w716 w728 w745 w761 w775]
        tunnel: w702 -> [w715 _ w744 w760 w774]
        frame "Generic" {
          w714 = refnum<vi> refnum  # 通用
          n211 = Variant To Data(type=w714, Variant=w715) -> (data=w713:refnum<vi>)  [unwired: 1 in, 1 out]
          n212 = property class="Gen"(reference=w713) -> ("ClassName"=w712:string)  [unwired: 1 in, 2 out]
          n213 = Format Into String(format string="%s (%s)", w716, w712) -> (resulting string=w719:string)  [unwired: 2 in, 1 out]
          n214 = Build Array(w724, w719) -> (w723:string[])
          n215 = invoke class="Tree" method="Edit Tree Items.Add Item"(reference=w725, "Parent Tag"=w727, "Child Position"=-1, "Left Cell"=w722, "Child Text"=w723, "Child Only?"=FALSE) -> (error out=w718:errorcluster, "Edit Tree Items:Add Item"=w717:string)  [unwired: 3 in, 7 out]
        }
        frame Default {
          n216 = Format Into String(format string="%s", w728) -> (resulting string=w731:string)  [unwired: 2 in, 1 out]
          n217 = Build Array(w736, w731) -> (w735:string[])
          n218 = invoke class="Tree" method="Edit Tree Items.Add Item"(reference=w737, "Parent Tag"=w739, "Child Position"=-1, "Left Cell"=w734, "Child Text"=w735, "Child Only?"=FALSE) -> (error out=w730:errorcluster, "Edit Tree Items:Add Item"=w729:string)  [unwired: 3 in, 7 out]
        }
        frame "LVObjVI" {
          n219 = Variant To Data(type=refnum<vi> refnum ("vi reference"), Variant=w744) -> (data=w743:refnum<vi>)  [unwired: 1 in, 1 out]
          n220 = property class="VI"(reference=w743) -> ("VIType"=w742:T6, "Name"=w741:string)  [unwired: 1 in, 2 out]
          n221 = Format Into String(format string="%s (%s, %s)", w745, w742, w741) -> (resulting string=w748:string)  [unwired: 2 in, 1 out]
          n222 = Build Array(w753, w748) -> (w752:string[])
          n223 = invoke class="Tree" method="Edit Tree Items.Add Item"(reference=w754, "Parent Tag"=w756, "Child Position"=-1, "Left Cell"=w751, "Child Text"=w752, "Child Only?"=FALSE) -> (error out=w747:errorcluster, "Edit Tree Items:Add Item"=w746:string)  [unwired: 3 in, 7 out]
        }
        frame "LVObjApp" {
          n224 = control-ref of="This Application"() -> (w757:refnum<vi>)
          n225 = Variant To Data(type=w757, Variant=w760) -> (data=w759:refnum<vi>)  [unwired: 1 in, 1 out]
          n226 = property class="App"(reference=w759) -> ("App.Name"=w758:string)  [unwired: 1 in, 2 out]
          n227 = Format Into String(format string="%s (%s)", w761, w758) -> (resulting string=w764:string)  [unwired: 2 in, 1 out]
          n228 = Build Array(w769, w764) -> (w768:string[])
          n229 = invoke class="Tree" method="Edit Tree Items.Add Item"(reference=w770, "Parent Tag"=w772, "Child Position"=-1, "Left Cell"=w767, "Child Text"=w768, "Child Only?"=FALSE) -> (error out=w763:errorcluster, "Edit Tree Items:Add Item"=w762:string)  [unwired: 3 in, 7 out]
        }
        frame "GenericClass" {
          n230 = call <vilib>:"GetLVClassInfo.vi"("Variant"=w774) -> ("LV Class File Name"=w773:string)  [unwired: 8 in, 2 out]
          n231 = Format Into String(format string="%s (%s)", w775, w773) -> (resulting string=w778:string)  [unwired: 2 in, 1 out]
          n232 = Build Array(w783, w778) -> (w782:string[])
          n233 = invoke class="Tree" method="Edit Tree Items.Add Item"(reference=w784, "Parent Tag"=w786, "Child Position"=-1, "Left Cell"=w781, "Child Text"=w782, "Child Only?"=FALSE) -> (error out=w777:errorcluster, "Edit Tree Items:Add Item"=w776:string)  [unwired: 3 in, 7 out]
        }
      }
    }
  }
  n234 = Unbundle By Name(w3) -> ("Traverse"=w5:bool)
  n235 = call "Colorize.vi"("Tag"=w2, "Type Descriptor Enum"=w1, "VariantTree in"=w3) -> ()  [unwired: 7 in, 2 out]
  n236 = case shown="真" w5 {
    tunnel: "Variant" -> [_ w797]
    tunnel: w2 -> [_ w794]
    tunnel: [w787 w793] -> w7
    tunnel: w3 -> [w787 w792]
    tunnel: w8 -> [w788 w791]
    tunnel: [w788 w790] -> w6
    frame False {
    }
    frame True {
      n237 = call <userlib>:"Get Variant Attributes__ogtk.vi"("error in"=w791, "Variant"=w797) -> ("error out"=w789:errorcluster, "value(s)"=w798:variant[], "names"=w796:string[])  [unwired: 2 in, 1 out]
      n238 = Array Size(array=w796) -> (size(s)=w795:i32)
      n239 = case shown="默认" w795 {
        tunnel: w789 -> [w799 w816]
        tunnel: w798 -> [_ w814]
        tunnel: w796 -> [_ w810]
        tunnel: w794 -> [_ w804]
        tunnel: w792 -> [w800 w803]
        tunnel: [w800 w809] -> w793
        tunnel: [w799 w815] -> w790
        frame 0 {
        }
        frame Default {
          # "Has Attributes"
          n240 = Unbundle By Name(w803) -> ("Tree Ref"=w802:refnum<vi>)
          n241 = invoke on="AddItem" class="Tree" method="Edit Tree Items.Add Item"(reference=w802, error in=w816, "Parent Tag"=w804, "Child Position"=-1, "Left Cell"="Attributes" ("Left Cell String")) -> (reference out=w801:refnum<vi>, error out=w813:errorcluster, "Edit Tree Items:Add Item"=w807:string)  [unwired: 4 in, 6 out]
          n242 = for {
            tunnel: w814 -> [w822] mode=indexing
            tunnel: [w819] -> w811 mode=indexing
            tunnel: w810 -> [w818] mode=indexing
            shift-right: [w820] -> w812
            shift-left: w813 -> [w821]
            n243 = call <userlib>:"Set Data Name__ogtk.vi"("error in (no error)"=w821, "Data Name"=w818, "Data"=w822) -> ("error out"=w820:errorcluster, "Renamed Data"=w819:variant)  [unwired: 7 in]
          }
          n244 = property class="Tree"(reference=w801, "Active Item Tag"=w807, "ActiveColNum"=0 ("Active Cell:Active Column Number"), "CellFontColor"=u32 11842740) -> ()  [unwired: 1 in, 2 out]
          n245 = call-dynamic "browseVariantArray.vi"("Array of Variants"=w811, "error in"=w812, "ParentTag"=w807, "VariantProbe.lvclass in"=w803) -> ("error out"=w815:errorcluster, "VariantProbe.lvclass out"=w809:refnum<class "VariantTree__VP.lvclass">)  [unwired: 4 in]
        }
      }
    }
  }
  "VariantProbe.lvclass out" <- w7
  "error out" <- w6
